vi "noisewave.vi"() -> ()   [LabVIEW 2016]
uses:
  <vilib>/express/express analysis/Spectral/Block/exnSpectralBlock spectral measurements RMS poly.vi
  <vilib>/express/express analysis/Spectral/Block/exnSpectralBlock spectral measurements RMS WFM.vi
  <vilib>/express/express analysis/Spectral/Block/exnSpectralBlock spectral measurements RMS DDT.vi
  <vilib>/express/express analysis/Spectral/XNode/ExpressSpectralMeasurementsBlockNode.xnode
  <vilib>/measure/NI_MABase.lvlib
panel:
  in  "Stop Button":bool
  out "FFT -RMS -2-":dynamicdata(graph)
  out "FFT-RMS-1-":cluster{"f0":dbl, "df":dbl, "magnitude":dbl[]}(graph)
  out "Waveform Graph":waveform(dbl)(graph)
  in  "seed":i32=-1
  in  "sampling info 2":cluster{"Fs":dbl, "#s":dbl}={"Fs"=1000.0, "#s"=1000.0} {"Fs" format="%.2p"}
  in  "standard deviation":dbl=1.0 format="%.2p"
  in  "signal type":T1(ring)
  in  "reset signal":bool
  in  "offset":dbl format="%0.2p"
  in  "sampling info":cluster{"Fs":dbl, "#s":dbl}={"Fs"=1000.0, "#s"=1000.0} {"Fs" format="%.2p"}
  in  "amplitude":dbl(knob)=1.0 scale=0.0..10.0
  in  "frequency":dbl=10.0 format="%0.2p"
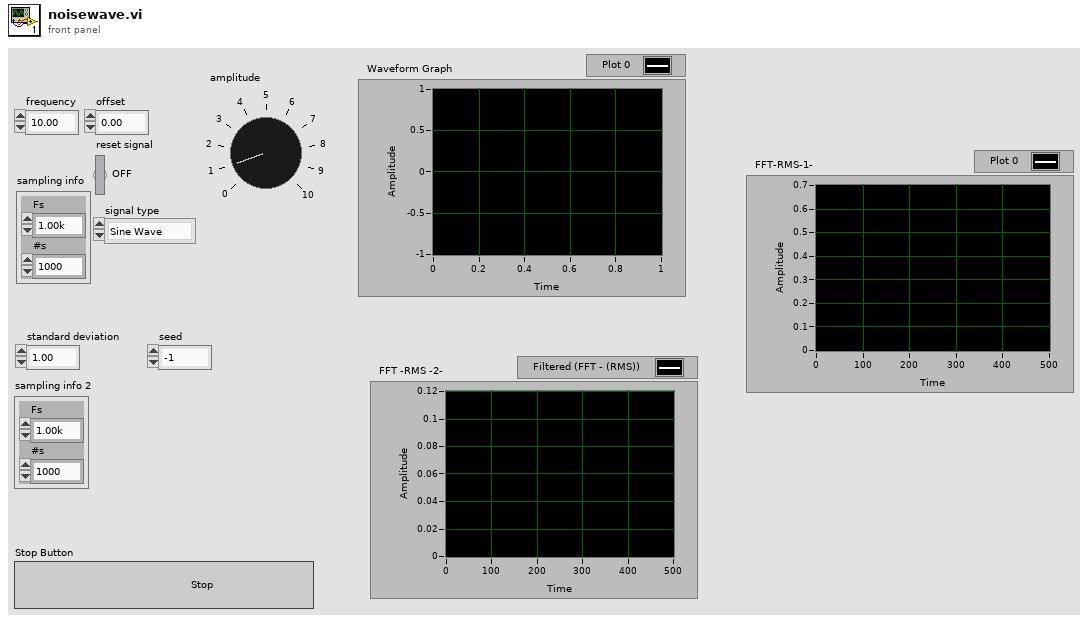
[diagram p1: front panel]
types:
  T1 = enum16{"Sine Wave", "Triangle Wave", "Square Wave", "Sawtooth Wave"}
  T2 = cluster{"averaging mode":u16, "weighting mode":u16, "number of averages":u32}
  T3 = cluster{"dB On (F)":bool, "unwrap phase (F)":bool, "convert to degree (F)":bool}
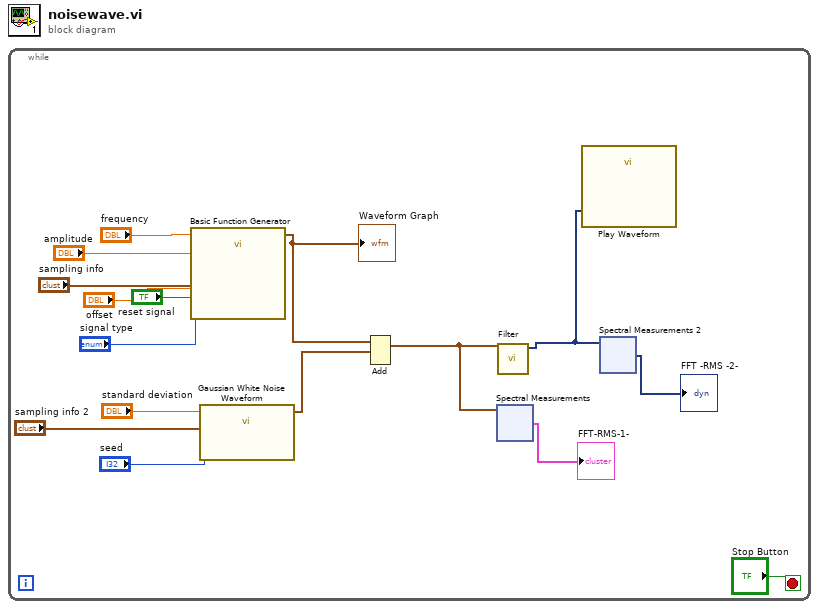
[diagram p0: block diagram]
diagram:
  n1 = while {
    stop <- "Stop Button" stop-if-true
    n2 = call <vilib>:"Basic Function Generator.vi"("offset"="offset", "reset signal"="reset signal", "sampling info"="sampling info", "signal type"="signal type", "amplitude"="amplitude", "frequency"="frequency") -> ("signal out"=w6:waveform(dbl))  [unwired: 3 in, 2 out]
    "Waveform Graph" <- w6
    n3 = call <vilib>:"Gaussian White Noise Waveform.vi"("sampling info"="sampling info 2", "seed"="seed", "standard deviation"="standard deviation") -> ("signal out"=w7:waveform(dbl))  [unwired: 7 in, 1 out]
    n4 = Add(1:w7, 2:w6) -> (0:w5:waveform(dbl))  [unwired: 1 in, 1 out]
    n5 = xnode "Spectral Measurements"("Signals"=w5) -> ("FFT - (RMS)"=→"FFT-RMS-1-":cluster{"f0":dbl, "df":dbl, "magnitude":dbl[]})  [unwired: 1 in, 2 out]
    n6 = call "Filter"("Signal"=w5) -> ("Filtered Signal"=w2:dynamicdata)  [unwired: 9 in, 1 out]
    n7 = call "Play Waveform"("Data"=w2) -> ()  [unwired: 18 in, 1 out]
    n8 = xnode "Spectral Measurements 2"("Signals"=w2) -> ("FFT - (RMS)"=→"FFT -RMS -2-":dynamicdata)  [unwired: 1 in, 2 out]
  }
